vi "Get Models for Type.vi"(8 "error in (no error)":errorcluster, 10 "Type":string, 11 "HAL Editor in":refnum<class "HAL Editor.lvclass">) -> (0 "error out":errorcluster, 1 "Models":string[](array[string]), 2 "Devices":refnum<class "Device.lvclass">[](array[class]), 3 "HAL Editor out":refnum<class "HAL Editor.lvclass">)   [LabVIEW 2012, in "HAL Config.lvlib" / "HAL Editor.lvclass"]
uses:
  HAL Editor.lvclass
  build/ppl/lv-hal.lvlibp/Device/Device.lvclass
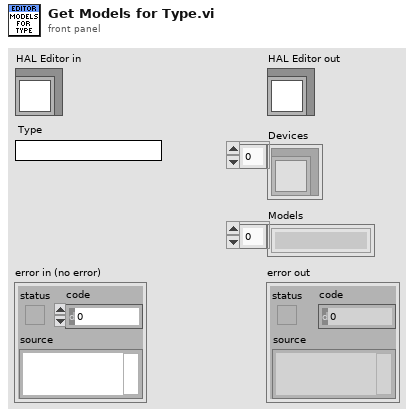
[diagram p1: front panel]
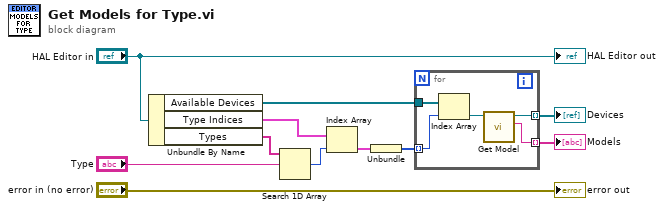
[diagram p0: block diagram]
diagram:
  n1 = Unbundle By Name("HAL Editor in") -> ("Available Devices"=w3:refnum<class "Device.lvclass">[], "Type Indices"=w9:cluster{"Indices":i32[]}[], "Types"=w10:string[])
  n2 = Search 1D Array(1D array=w10, element="Type") -> (index of element=w8:i32)  [unwired: 1 in]
  n3 = Index Array(array=w9, index=w8) -> (element=w5:cluster{"Indices":i32[]})
  n4 = Unbundle(w5) -> ("Indices"=w4:i32[])
  n5 = for {
    tunnel: w4 -> [w15] mode=indexing
    tunnel: w3 -> [w16]
    tunnel: [w13] -> w2 mode=indexing
    tunnel: [w12] -> w1 mode=indexing
    n6 = Index Array(array=w16, index=w15) -> (element=w14:refnum<class "Device.lvclass">)
    n7 = call-dynamic "Get Model.vi"("Device in"=w14) -> ("Model"=w12:string, "Device out"=w13:refnum<class "Device.lvclass">)  [unwired: 8 in, 1 out]
  }
  "Devices" <- w2
  "Models" <- w1
  "error out" <- "error in (no error)"
  "HAL Editor out" <- "HAL Editor in"
